vi "Log of Magnitude Square.vi"(5 "Real":fxp<+/-,16,1> format="%.16g", 7 "Imaginary":fxp<+/-,16,1> format="%.16g", 9 "Input Valid":bool=TRUE) -> (6 "Log Magnitude":fxp<+/-,34,12> format="%.26g", 8 "Output Valid":bool)   [LabVIEW 2011]
doc: "This VI calculates 10*Log (Magnitude(Z)^2).\n\n\n<b> Latency = 17 Ticks </b>"
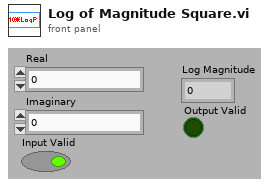
[diagram p1: front panel]
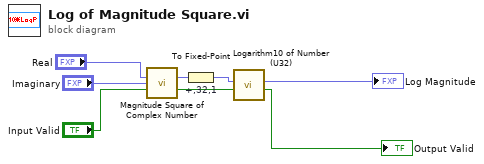
[diagram p0: block diagram]
diagram:
  n1 = call "Magnitude Square of Complex Number.vi"("Real"="Real", "Imaginary"="Imaginary", "Input Valid"="Input Valid") -> ("Magnitude^2"=w7:fxp<+,48,14>, "Output Valid"=w8:bool)  [unwired: 11 in]
  n2 = To Fixed-Point "+,32,1"(number=w7) -> (fixed-point=w6:fxp<+,32,1>)  [unwired: 1 in]
  n3 = call <userlib>:"Logarithm10 of Number (U32).vi"("Input Valid"=w8, "Input Number (0.32)"=w6) -> ("Output Valid"=→"Output Valid":bool, "Logarithm"=→"Log Magnitude":fxp<+/-,34,12>)  [unwired: 6 in, 2 out]
